vi "UART Run.vi"(0 "UART Driver in":refnum<class "UART Driver.lvclass">, 11 "error in":errorcluster) -> (4 "UART Driver out":refnum<class "UART Driver.lvclass">, 15 "error out":errorcluster)   [LabVIEW 2012, in "UART_Host_Driver.lvlib" / "UART Driver.lvclass"]
doc: "Start the execution of UART FPGA personality."
uses:
  UART Driver.lvclass
  Typedefs/FPGA VI Reference.ctl
  UART Driver.lvclass/UART Driver.ctl
  <vilib>/FPGAPlugInAG/Dynamic/niLvFpga_Run_Dynamic.vi
  <vilib>/rvi/interface/nirviMethod/nirviMethod.xnode
  UART_Host_Driver.lvlib
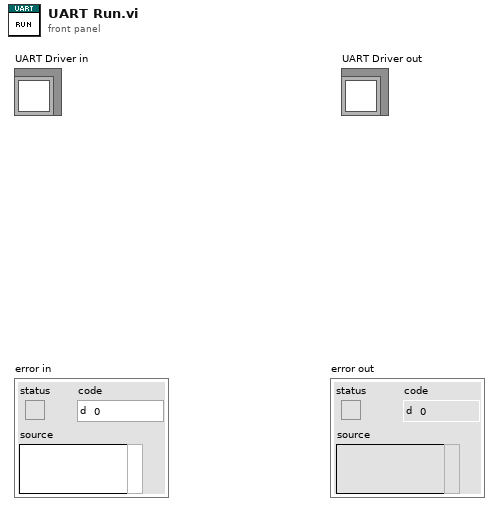
[diagram p1: front panel]
types:
  T1 = typedef "UART_Host_Driver.lvlib/FPGA VI Reference.ctl" = refnum<k20>
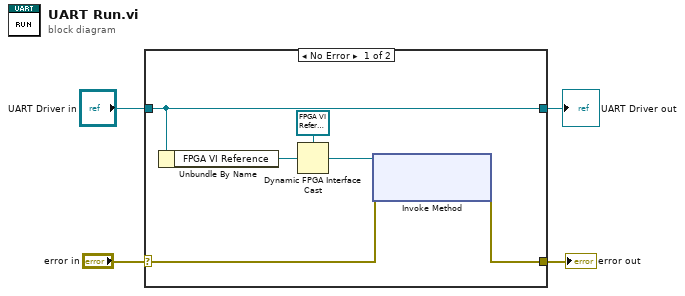
[diagram p0: block diagram]
diagram:
  n1 = case shown="No Error" "error in" {
    selector: "error in" -> [w7 w12]
    tunnel: [w5 w12] -> w3
    tunnel: [w6 w11] -> w2
    tunnel: "UART Driver in" -> [w6 w11]
    frame No Error {
      n2 = Unbundle By Name(w6) -> ("FPGA VI Reference"=w10:refnum<k20>)
      n3 = Dynamic FPGA Interface Cast(Session In=T1 refnum ("FPGA VI Reference"), Type=w10) -> (Session Out=w8:T1)
      n4 = xnode "Invoke Method"("FPGA VI Reference In"=w8, "error in"=w7) -> ("error out"=w5:errorcluster)  [unwired: 1 in, 1 out]
    }
    frame Error {
    }
  }
  "error out" <- w3
  "UART Driver out" <- w2
